vi "get sort histo data.vi"(8 "error IO":errorcluster, 10 "Pixie input array 2":u16[](array[numeric])=array[250000 elements], 11 "listmodedata in":u16[](array[numeric])=array[250000 elements]) -> (0 "error out":errorcluster, 1 "channel 0-4 time out":u16[][](array[numeric]), 2 "Sum of gated counts":i32=1521, 3 "channel 0-4 energy out":u16[][](array[numeric]))   [LabVIEW 2016]
doc: "This vi inputslist mode data and creates 4 1d histograms of the gated pixie data"
panel:
  in  "scale factor":dbl=1.0
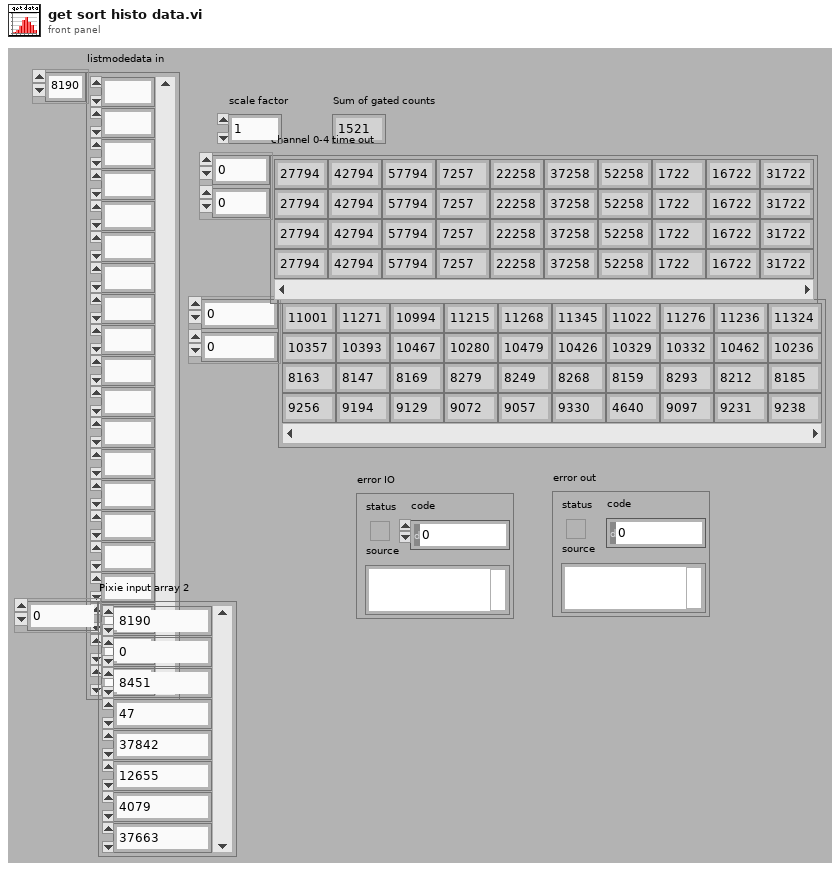
[diagram p1: front panel]
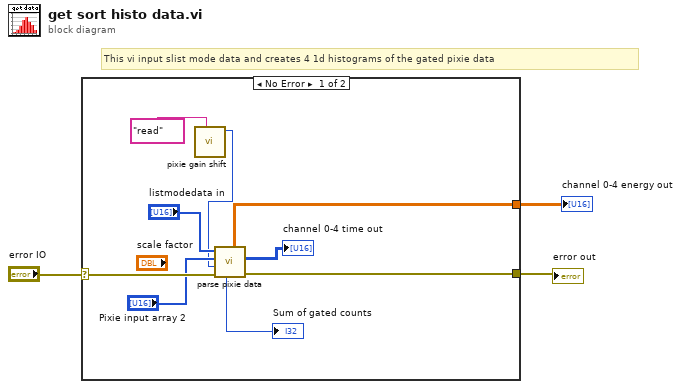
[diagram p0: block diagram]
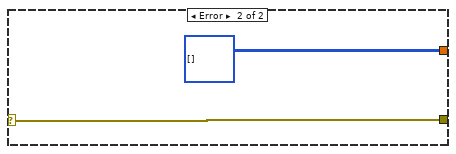
[diagram p2: hidden frame]
diagram:
  # "This vi input slist mode data and creates 4 1d histograms of the gated pixie data"
  n1 = case shown="No Error" "error IO" {
    selector: "error IO" -> [w12 w14]
    tunnel: [w9 w14] -> w3
    tunnel: [w8 i32[][] [] ("sum Histogram out channel 0")] -> w1
    frame No Error {
      n2 = call "pixie gain shift.vi"("shift control"="read") -> ("gain out"=w4:i32)  [unwired: 10 in]
      n3 = call "parse pixie data.vi"("error in (no error)"=w12, "scale factor"=w4, "Pixie input array 2"="Pixie input array 2", "Pixie input array"="listmodedata in") -> ("error out"=w9:errorcluster, "time 0-3"=→"channel 0-4 time out":u32[][], "0-3 events"=w8:dbl[][], "Sum of gated counts"=→"Sum of gated counts":i32)  [unwired: 3 in, 1 out]
    }
    frame Error {
    }
  }
  "error out" <- w3
  "channel 0-4 energy out" <- w1
